vi "P3060_获得设备属性.vi"(8 "错误输入（无错误）":errorcluster, 11 "句柄输入":i32) -> (0 "错误输出":errorcluster, 2 "板卡属性":T1 {"厂商ID" format="%x"; "设备ID" format="%x"}, 3 "句柄输出":i32)   [LabVIEW 2010]
doc: "获得设备属性。"
uses:
  _SubVI/dll/P3060.dll
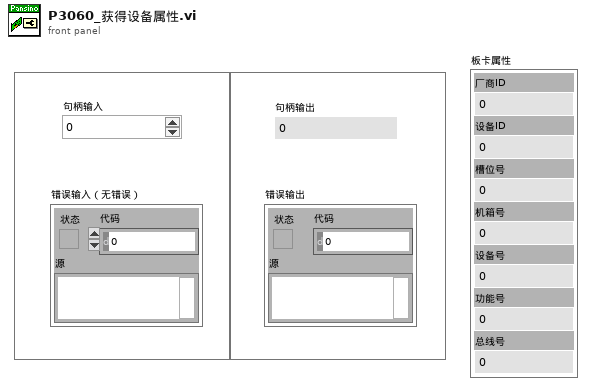
[diagram p1: front panel]
types:
  T1 = cluster{"厂商ID":u16, "设备ID":u16, "槽位号":i16, "机箱号":i16, "设备号":u16, "功能号":u16, "总线号":u16}
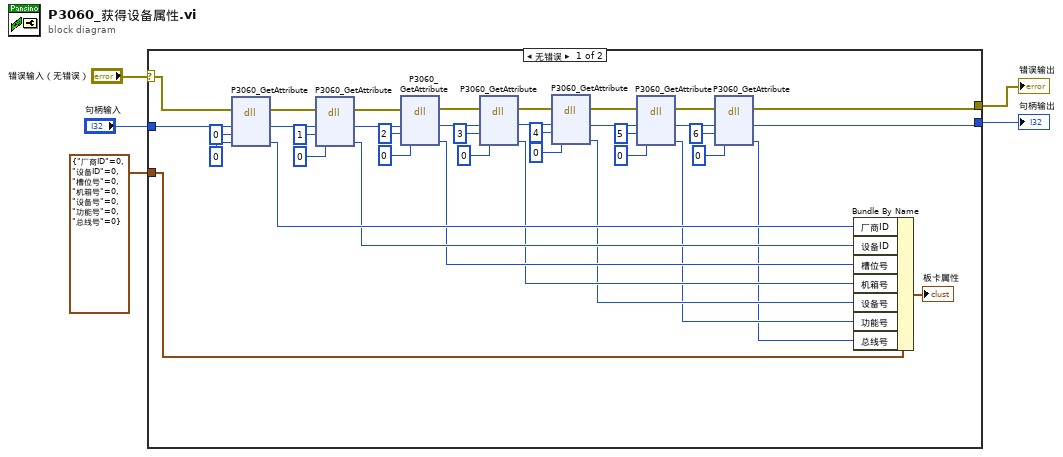
[diagram p0: block diagram]
diagram:
  n1 = case shown="无错误" "错误输入（无错误）" {
    selector: "错误输入（无错误）" -> [w44 w46]
    tunnel: [w8 w46] -> w4
    tunnel: "句柄输入" -> [w43 w45]
    tunnel: T1 {"厂商ID"=0, "设备ID"=0, "槽位号"=0, "机箱号"=0, "设备号"=0, "功能号"=0, "总线号"=0} -> [w23 _]
    tunnel: [w7 w45] -> w1
    frame No Error {
      n2 = dll-call lib="D:/driver/trunk/Drivers/P3060/P3060API/P3060APILV/Labview/P3060/_SubVI/dll/P3060.dll" fn="P3060_GetAttribute"(error in=w44, "hDev"=w43, "Attribute"=u32 0, "attrstate"=u16 0) -> (error out=w41:errorcluster, "hDev"=w40:i32, "attrstate"=w22:u16)  [unwired: 4 in, 1 out]
      n3 = dll-call lib="D:/driver/trunk/Drivers/P3060/P3060API/P3060APILV/Labview/P3060/_SubVI/dll/P3060.dll" fn="P3060_GetAttribute"(error in=w41, "hDev"=w40, "Attribute"=u32 1, "attrstate"=u16 0) -> (error out=w38:errorcluster, "hDev"=w37:i32, "attrstate"=w21:u16)  [unwired: 4 in, 1 out]
      n4 = dll-call lib="D:/driver/trunk/Drivers/P3060/P3060API/P3060APILV/Labview/P3060/_SubVI/dll/P3060.dll" fn="P3060_GetAttribute"(error in=w38, "hDev"=w37, "Attribute"=u32 2, "attrstate"=i16 0) -> (error out=w35:errorcluster, "hDev"=w34:i32, "attrstate"=w20:i16)  [unwired: 4 in, 1 out]
      n5 = dll-call lib="D:/driver/trunk/Drivers/P3060/P3060API/P3060APILV/Labview/P3060/_SubVI/dll/P3060.dll" fn="P3060_GetAttribute"(error in=w35, "hDev"=w34, "Attribute"=u32 3 ("hDev"), "attrstate"=i16 0) -> (error out=w32:errorcluster, "hDev"=w31:i32, "attrstate"=w19:i16)  [unwired: 4 in, 1 out]
      n6 = dll-call lib="D:/driver/trunk/Drivers/P3060/P3060API/P3060APILV/Labview/P3060/_SubVI/dll/P3060.dll" fn="P3060_GetAttribute"(error in=w32, "hDev"=w31, "Attribute"=u32 4, "attrstate"=u16 0) -> (error out=w29:errorcluster, "hDev"=w28:i32, "attrstate"=w18:u16)  [unwired: 4 in, 1 out]
      n7 = dll-call lib="D:/driver/trunk/Drivers/P3060/P3060API/P3060APILV/Labview/P3060/_SubVI/dll/P3060.dll" fn="P3060_GetAttribute"(error in=w29, "hDev"=w28, "Attribute"=u32 5, "attrstate"=u16 0) -> (error out=w26:errorcluster, "hDev"=w25:i32, "attrstate"=w17:u16)  [unwired: 4 in, 1 out]
      n8 = dll-call lib="D:/driver/trunk/Drivers/P3060/P3060API/P3060APILV/Labview/P3060/_SubVI/dll/P3060.dll" fn="P3060_GetAttribute"(error in=w26, "hDev"=w25, "Attribute"=u32 6, "attrstate"=u16 0) -> (error out=w8:errorcluster, "hDev"=w7:i32, "attrstate"=w16:u16)  [unwired: 4 in, 1 out]
      n9 = Bundle By Name(cluster=w23, "厂商ID"=w22, "设备ID"=w21, "槽位号"=w20, "机箱号"=w19, "设备号"=w18, "功能号"=w17, "总线号"=w16) -> (→"板卡属性":T1)
    }
    frame Error {
    }
  }
  "错误输出" <- w4
  "句柄输出" <- w1
